vi "Filter Plugin by Version.vi"(10 "Version Filter":T2, 11 "Discovered Plugins":T1[](array[typedef])) -> (2 "Match found":bool, 3 "Matching Plugin":T1)   [LabVIEW 2021, in "CIFPluginManager.lvclass"]
uses:
  CIFPluginManager.lvclass
  Common/typedef/Discovered Plugin.ctl
  <vilib>/CIF Foundation/CIF Core/CIFCore/Common/Typedef/Version.ctl
  Common/typedef/Plugin Metadata.ctl
  Common/typedef/Loader Type.ctl
  CIFPluginManager.lvclass/CIFPluginManager.ctl
  <vilib>/CIF Foundation/CIF Core/CIFCore/Common/CIFCoreCommon.lvlib
  Common/Manager Common.lvlib
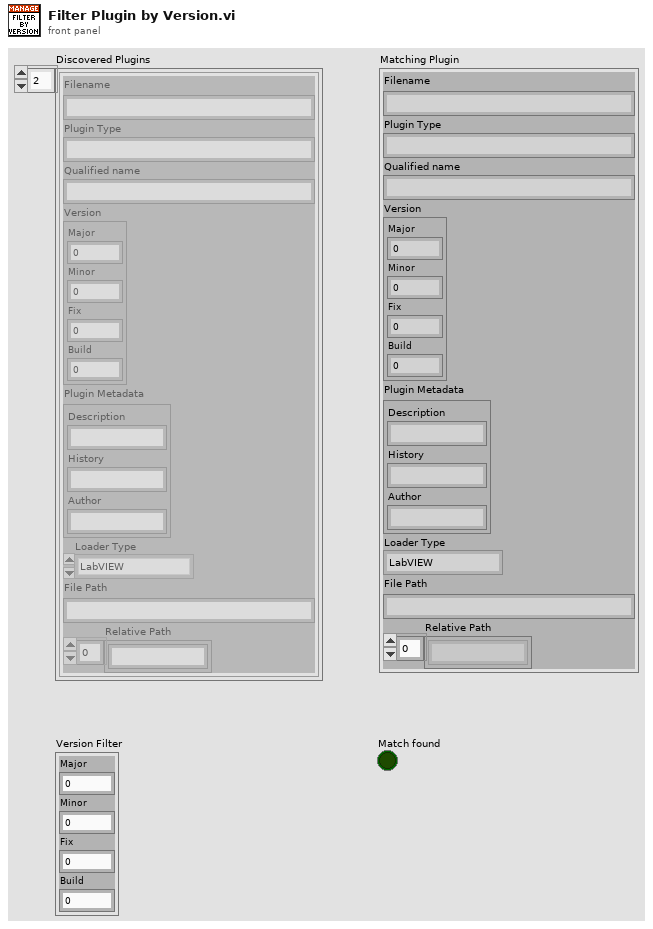
[diagram p1: front panel]
types:
  T1 = typedef "Manager Common.lvlib/Discovered Plugin.ctl" = cluster{"Filename":string, "Plugin Type":string, "Qualified name":string, "Version":T2, "Plugin Metadata":T3, "Loader Type":T4, "File Path":string, "Relative Path":string[]}
  T2 = typedef "CIFCoreCommon.lvlib/Version.ctl" = cluster{"Major":i32, "Minor":i32, "Fix":i32, "Build":i32}
  T3 = typedef "Manager Common.lvlib/Plugin Metadata.ctl" = cluster{"Description":string, "History":string, "Author":string}
  T4 = typedef "Manager Common.lvlib/Loader Type.ctl" = enum16{"LabVIEW"}
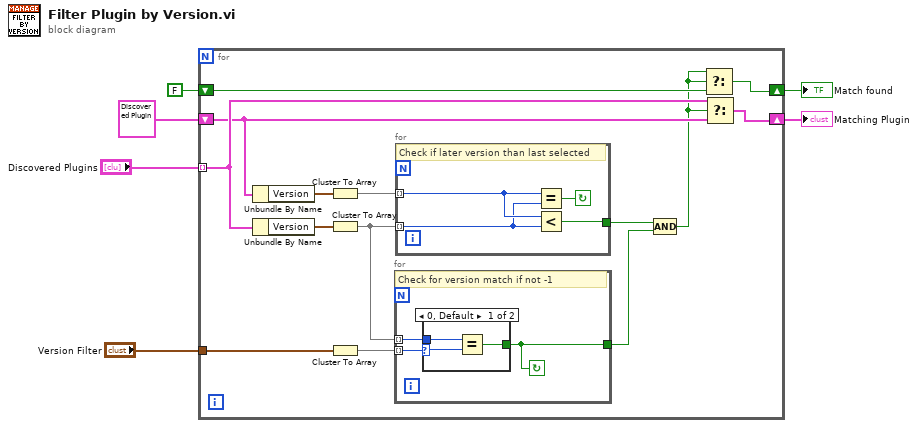
[diagram p0: block diagram]
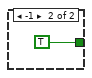
[diagram p2: hidden frame]
diagram:
  n1 = for {
    tunnel: "Discovered Plugins" -> [w17] mode=indexing
    tunnel: "Version Filter" -> [w19]
    shift-right: [w12] -> w3
    shift-left: T1 {"Filename"="", "Plugin Type"="", "Qualified name"="", "Version"={"Major"=0, "Minor"=0, "Fix"=0, "Build"=0}, "Plugin Metadata"={"Description"="", "History"="", "Author"=""}, "Loader Type"=enum."LabVIEW", "File Path"="", "Relative Path"=[]} ("Discovered Plugin") -> [w15]
    shift-right: [w9] -> w1
    shift-left: FALSE -> [w8]
    n2 = Unbundle By Name(w15) -> ("Version"=w16:T2)
    n3 = Unbundle By Name(w17) -> ("Version"=w20:T2)
    n4 = Cluster To Array(cluster=w16) -> (array=w14:i32[])
    n5 = Cluster To Array(cluster=w20) -> (array=w10:i32[])
    n6 = Cluster To Array(cluster=w19) -> (array=w18:i32[])
    n7 = for {
      tunnel: w18 -> [w27] mode=indexing
      tunnel: w10 -> [w26] mode=indexing
      tunnel: [w25] -> w13
      stop <- w25 continue-if-true
      # "Check for version match if not -1"
      n8 = case shown="0, Default" w27 {
        selector: w27 -> [w30 _]
        tunnel: w26 -> [w28 _]
        tunnel: [w29 TRUE] -> w25
        frame 0, Default {
          n9 = Equal?(x=w28, y=w30) -> (x = y?=w29:bool)
        }
        frame -1 {
        }
      }
    }
    n10 = for {
      tunnel: w10 -> [w22] mode=indexing
      tunnel: w14 -> [w23] mode=indexing
      tunnel: [w24] -> w11
      stop <- w21 continue-if-true
      # "Check if later version than last selected"
      n11 = Equal?(x=w23, y=w22) -> (x = y?=w21:bool)
      n12 = Less?(x=w23, y=w22) -> (x < y?=w24:bool)
    }
    n13 = Compound Arithmetic op=AND(w11, w13) -> (w7:bool)
    n14 = Select(t=w7, s=w7, f=w8) -> (s? t:f=w9:bool)
    n15 = Select(t=w17, s=w7, f=w15) -> (s? t:f=w12:T1)
  }
  "Matching Plugin" <- w3
  "Match found" <- w1
